vi "Calculate Number of Rows and Columns.vi"(9 "# of items":i32, 11 "Container Bounds":T1) -> (1 "# of Columns":i32, 2 "# of Rows":i32, 3 "Cell Bounds":T1)   [LabVIEW 2011]
doc: "For the given container bounds, find the Rows/Columns that provide the smallest aspect ratio so that thumbnails are as close to a square as possible."
uses:
  <vilib>/Utility/miscctls.llb/LVBoundsTypeDef.ctl
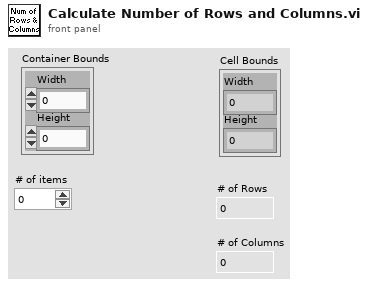
[diagram p1: front panel]
types:
  T1 = typedef "LVBoundsTypeDef.ctl" = cluster{"Width":u32, "Height":u32}
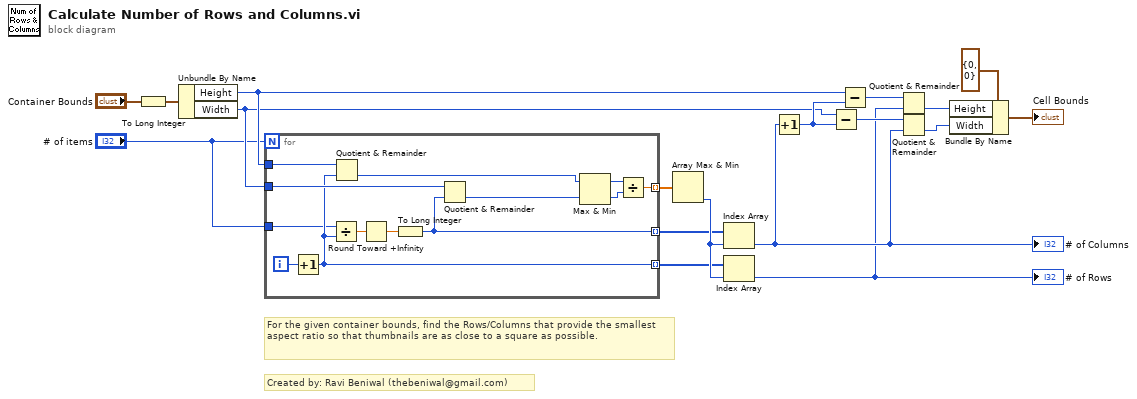
[diagram p0: block diagram]
diagram:
  # "For the given container bounds, find the Rows/Columns that provide the smallest aspect ratio so that thumbnails are as close to a square as possible."
  # "Created by: Ravi Beniwal (thebeniwal@gmail.com)"
  n1 = To Long Integer(number="Container Bounds") -> (32bit integer=w4:cluster{"Width":i32, "Height":i32})
  n2 = Unbundle By Name(w4) -> ("Height"=w3:i32, "Width"=w2:i32)
  n3 = for {
    N: "# of items" -> [_]
    tunnel: w3 -> [w31]
    tunnel: w2 -> [w30]
    tunnel: [w22] -> w15 mode=indexing
    tunnel: [w21] -> w17 mode=indexing
    tunnel: [w20] -> w16 mode=indexing
    tunnel: "# of items" -> [w19]
    i -> [w29]
    n4 = Increment(x=w29) -> (x+1=w21:i32)
    n5 = Divide(x=w19, y=w21) -> (x/y=w28:dbl)
    n6 = Quotient & Remainder(x=w31, y=w21) -> (floor(x/y)=w26:i32)  [unwired: 1 out]
    n7 = Round Toward +Infinity(x=w28) -> (ceil(x): smallest int >= x=w27:dbl)
    n8 = To Long Integer(number=w27) -> (32bit integer=w20:i32)
    n9 = Quotient & Remainder(x=w30, y=w20) -> (floor(x/y)=w25:i32)  [unwired: 1 out]
    n10 = Max & Min(x=w26, y=w25) -> (max(x,y)=w24:i32, min(x,y)=w23:i32)
    n11 = Divide(x=w24, y=w23) -> (x/y=w22:dbl)
  }
  n12 = Array Max & Min(array=w15) -> (min index (indices)=w18:i32)  [unwired: 3 out]
  n13 = Index Array(array=w16, index=w18) -> (element=w8:i32)
  "# of Columns" <- w8
  n14 = Index Array(array=w17, index=w18) -> (element=w6:i32)
  "# of Rows" <- w6
  n15 = Increment(x=w8) -> (x+1=w9:i32)
  n16 = Subtract(x=w2, y=w9) -> (x-y=w11:i32)
  n17 = Subtract(x=w3, y=w9) -> (x-y=w10:i32)
  n18 = Quotient & Remainder(x=w10, y=w6) -> (floor(x/y)=w13:i32)  [unwired: 1 out]
  n19 = Quotient & Remainder(x=w11, y=w8) -> (floor(x/y)=w12:i32)  [unwired: 1 out]
  n20 = Bundle By Name(cluster=T1 {"Width"=0, "Height"=0} ("Container Bounds"), "Height"=w13, "Width"=w12) -> (→"Cell Bounds":T1)
